vi "convert data to scan line array.vi"(6 "Fetch vector in":dbl[][](array[numeric]), 8 "Max":dbl, 9 "Min":dbl, 10 "Number of records":i32, 11 "error in (no error)":errorcluster) -> (2 "Hilbert out":dbl[][](array[numeric]), 3 "Scan array out":dbl[](array[numeric]))   [LabVIEW 2014]
uses:
  <vilib>/Analysis/NI_AALPro.lvlib
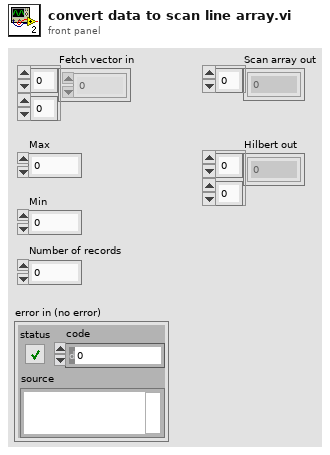
[diagram p1: front panel]
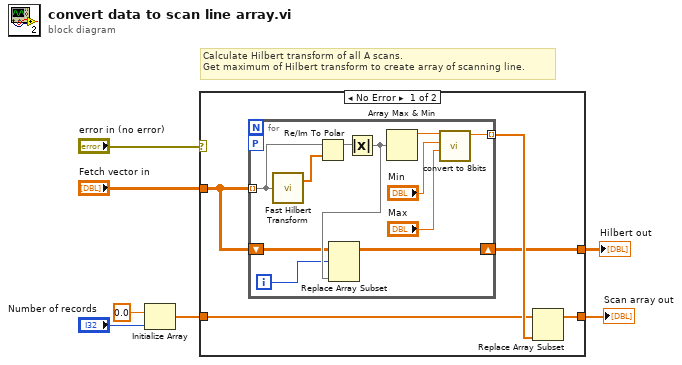
[diagram p0: block diagram]
diagram:
  # "Calculate Hilbert transform of all A scans. \nGet maximum of Hilbert transform to create array of scanning line."
  n1 = Initialize Array(0.0 ("element"), "Number of records") -> (w2:dbl[])
  n2 = case shown="No Error" "error in (no error)" {
    tunnel: "Fetch vector in" -> [w9 w24]
    tunnel: w2 -> [w11 w25]
    tunnel: [w10 w25] -> w6
    tunnel: [w8 w24] -> w1
    frame No Error {
      n3 = for {
        tunnel: w9 -> [w19] mode=indexing
        tunnel: [w20] -> w12 mode=indexing
        workers-P: _ -> [_]
        shift-right: [w14] -> w8
        shift-left: w9 -> [w15]
        i -> [w13]
        n4 = call <vilib>:"Fast Hilbert Transform.vi"("X"=w19) -> ("Hilbert{X}"=w17:dbl[])  [unwired: 1 out]
        n5 = Re/Im To Polar(2:w17, 3:w19) -> (1:w18:dbl[])  [unwired: 1 out]
        n6 = Absolute Value(x=w18) -> (abs(x)=w16:dbl[])
        n7 = Replace Array Subset(array=w15, new element=w16, index (row)=w13) -> (w14:dbl[][])  [unwired: 1 in]
        n8 = Array Max & Min(array=w16) -> (max value=w23:dbl)  [unwired: 3 out]
        n9 = call "convert to 8bits.vi"("max"="Max", "min"="Min", "input"=w23) -> ("output_8b"=w20:dbl)  [unwired: 8 in]
      }
      n10 = Replace Array Subset(array=w11, new element=w12) -> (w10:dbl[])  [unwired: 1 in]
    }
    frame Error {
    }
  }
  "Scan array out" <- w6
  "Hilbert out" <- w1
